vi "clFile_readFromFile.vi"(10 "file (use dialog)":path) -> (2 "clFileReader.lvclass":refnum<class "clFileReader.lvclass">, 3 "clFile.lvclass":refnum<class "clFile.lvclass">)   [LabVIEW 2016, in "vi_lib.lvlib" / "clFile.lvclass"]
uses:
  clFile.lvclass
  clFileReader/clFileReader.lvclass
  clFile.lvclass/clFile.ctl
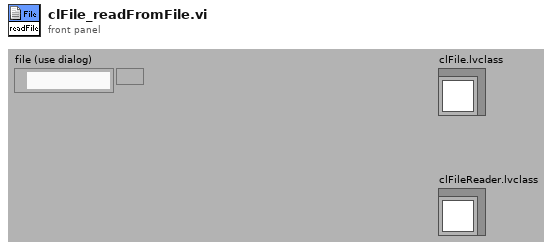
[diagram p1: front panel]
types:
  T1 = enum16{"open", "replace", "create", "open or create", "replace or create", "replace or create with confirmation"}
  T2 = enum16{"deny read/write", "deny write-only", "deny none"}
  T3 = enum16{"big-endian, network order", "native, host order", "little-endian"}
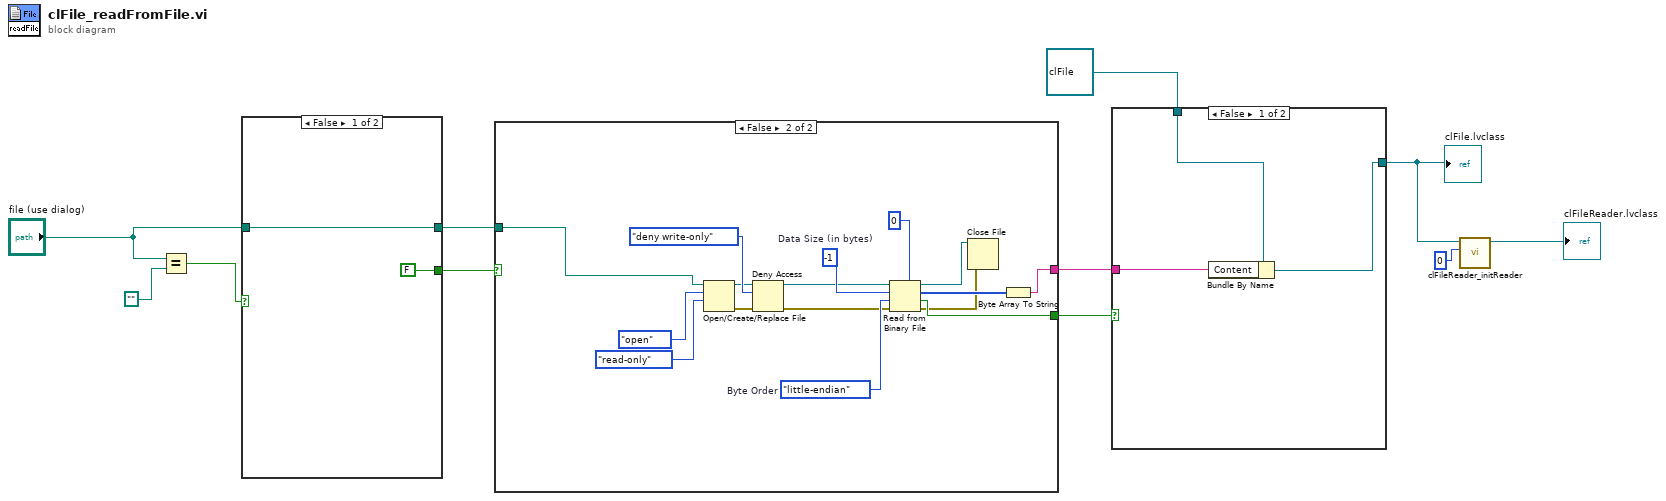
[diagram p0: block diagram]
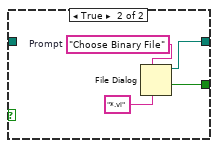
[diagram p2: hidden frame]
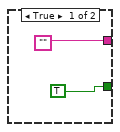
[diagram p3: hidden frame]
diagram:
  n1 = Equal?(x="file (use dialog)", y=path "") -> (x = y?=w8:bool)
  n2 = case shown="False" w8 {
    tunnel: [w13 w16] -> w6
    tunnel: "file (use dialog)" -> [w13 _]
    tunnel: [FALSE ("cancelled") w15] -> w5
    frame False {
    }
    frame True {
      w14 = "Choose Binary File"  # Prompt
      n3 = File Dialog(6:"*.vi" ("pattern (all files)"), 7:w14) -> (1:w15:bool, 3:w16:path)  [unwired: 1 in, 6 out]
    }
  }
  n4 = case shown="False" w5 {
    tunnel: [TRUE ("cancelled") w27] -> w10
    tunnel: ["" w23] -> w9
    tunnel: w6 -> [_ w22]
    frame True {
    }
    frame False {
      w29 = T3."little-endian"  # Byte Order
      w35 = i64 -1  # Data Size (in bytes)
      n5 = Open/Create/Replace File(file path (use dialog)=w22, operation (0:open)=T1."open", access (0:read/write)=enum16{"read/write", "read-only", "write-only"}."read-only") -> (refnum out=w31:refnum<file>, error out=w30:errorcluster)  [unwired: 1 in, 3 out]
      n6 = Deny Access(4:w30, 6:T2."deny write-only" ("deny mode (0:deny read/write)"), 7:w31) -> (0:w26:errorcluster, 3:w34:refnum<file>)
      n7 = Read from Binary File(5:u8 0, 8:w26, 9:w29, 10:w35, 11:w34) -> (0:w20:errorcluster, 1:w27:bool, 2:w24:u8[], 3:w21:refnum<file>)  [unwired: 1 out]
      n8 = Close File(refnum=w21, error in=w20) -> ()  [unwired: 2 out]
      n9 = Byte Array To String(unsigned byte array=w24) -> (string=w23:string)
    }
  }
  n10 = case shown="False" w10 {
    tunnel: w9 -> [w38 _]
    tunnel: refnum<class "clFile.lvclass"> refnum ("clFile.lvclass") -> [w37 w39]
    tunnel: [w36 w39] -> w3
    frame False {
      n11 = Bundle By Name(cluster=w37, "Content"=w38) -> (w36:refnum<class "clFile.lvclass">)
    }
    frame True {
    }
  }
  "clFile.lvclass" <- w3
  n12 = call "clFileReader_initReader.vi"("HiddenOffset"=u32 0, "clFile.lvclass"=w3) -> ("clFileReader.lvclass"=→"clFileReader.lvclass":refnum<class "clFileReader.lvclass">)  [unwired: 1 in, 8 out]
